vi "TDTSyn-Wait For Block.vi"(0 "IP Address":string, 5 "Port":i32, 9 "Timeout (s)":i32=10, 11 "error in (no error)":errorcluster, 12 "byte order":T1(ring)=enum."native, host order") -> (15 "error out":errorcluster)   [LabVIEW 2020]
panel:
  out "block name":string
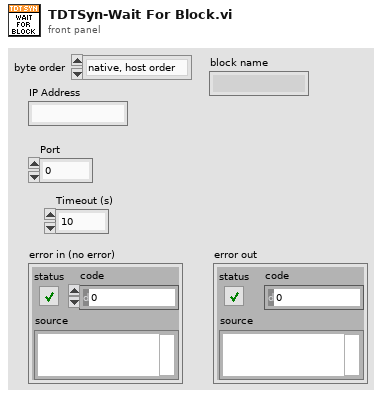
[diagram p1: front panel]
types:
  T1 = enum16{"big-endian, network order", "native, host order", "little-endian"}
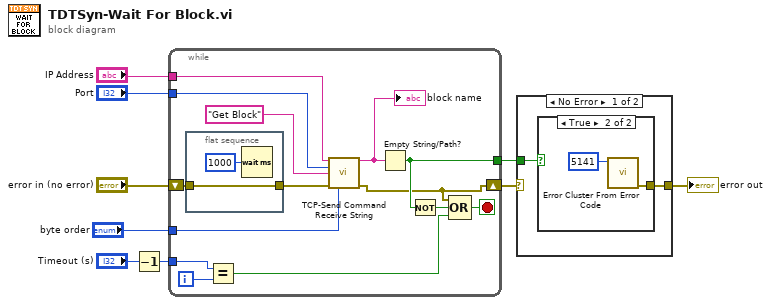
[diagram p0: block diagram]
diagram:
  n1 = Decrement(x="Timeout (s)") -> (x-1=w5:i32)
  n2 = while {
    shift-right: [w14] -> w4
    shift-left: "error in (no error)" -> [w12]
    tunnel: "IP Address" -> [w22]
    tunnel: "Port" -> [w23]
    tunnel: [w18] -> w2
    tunnel: w5 -> [w13]
    tunnel: "byte order" -> [w10]
    i -> [w19]
    stop <- w15 stop-if-true
    n3 = flat-sequence {
      tunnel: w12 -> [w25]
      tunnel: [w25] -> w11
      frame #0 {
        n4 = Wait (ms)(milliseconds to wait=u32 1000) -> ()  [unwired: 1 out]
      }
    }
    n5 = Equal?(x=w13, y=w19) -> (x = y?=w16:bool)
    n6 = call "TCP-Send Command Receive String.vi"("PXI Address"=w22, "Port"=w23, "Command"="Get Block", "error in (no error)"=w11, "byte order"=w10) -> ("data"=w20:string, "error out"=w14:errorcluster)  [unwired: 9 in]
    "block name" <- w20
    n7 = Empty String/Path?(string/path=w20) -> (empty?=w18:bool)
    n8 = Not(x=w18) -> (.not. x?=w17:bool)
    n9 = Compound Arithmetic op=OR(w14, w17, w16) -> (w15:bool)
  }
  n10 = case shown="No Error" w4 {
    selector: w4 -> [_ w30]
    tunnel: [w26 w30] -> w3
    tunnel: w2 -> [w27 _]
    frame No Error {
      n11 = case shown="True" w27 {
        tunnel: [_ w29] -> w26
        frame False {
        }
        frame True {
          n12 = call <vilib>:"Error Cluster From Error Code.vi"("error code (0)"=5141) -> ("error out"=w29:errorcluster)  [unwired: 8 in]
        }
      }
    }
    frame Error {
    }
  }
  "error out" <- w3
